vi "code2.vi"() -> ()   [LabVIEW 2019]
panel:
  in  "B":dbl
  out "Product":dbl
  out "Waveform Chart":dbl(graph)
  in  "A":dbl
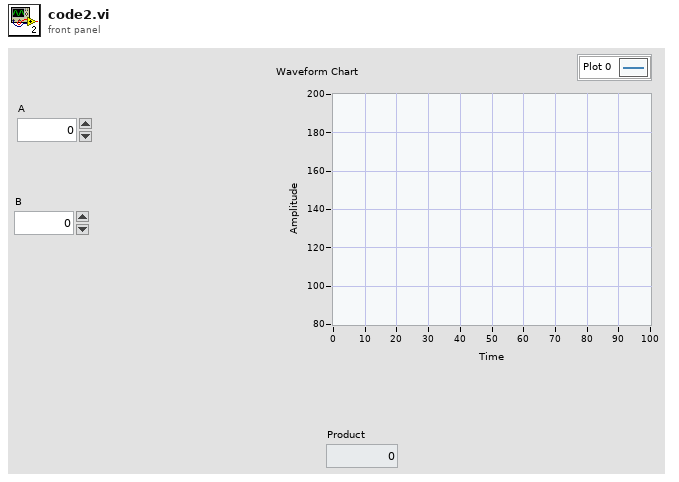
[diagram p1: front panel]
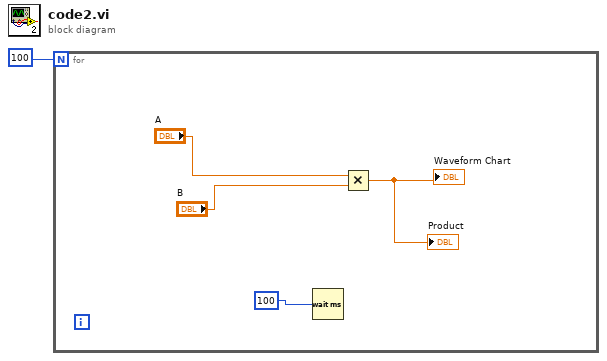
[diagram p0: block diagram]
diagram:
  n1 = for {
    N: 100 -> [_]
    n2 = Wait (ms)(milliseconds to wait=100) -> ()  [unwired: 1 out]
    n3 = Multiply(x="A", y="B") -> (x*y=→"Waveform Chart" →"Product":dbl)
  }
